vi "NanotecSMCPDDriver.create write string.vi"(1 "contollerID":i32, 3 "commandString":string, 5 "error in (no error)":errorcluster) -> (15 "writeString":string, 17 "expextedReturnString":string, 19 "error out":errorcluster)   [LabVIEW 2014, in "NanotecSMCPDDriver.lvlib"]
doc: "Composes the string, that will be written to the serial interface.\n\nTo access an individual controller, the controllerID must be in the range 1..254.\nTo select all controllers, the controllerID must equal -2."
uses:
  NanotecSMCPDDriver.lvlib
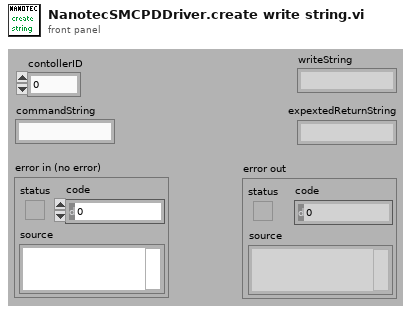
[diagram p1: front panel]
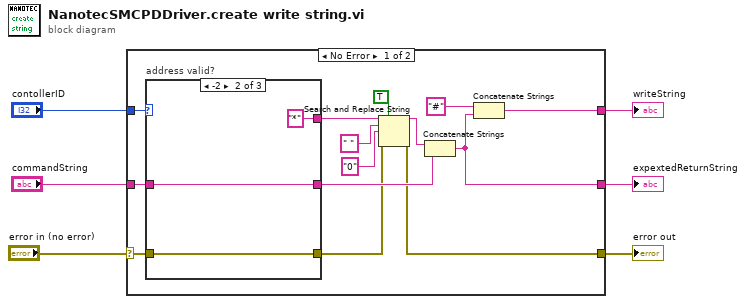
[diagram p0: block diagram]
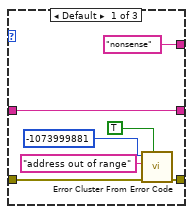
[diagram p2: hidden frame]
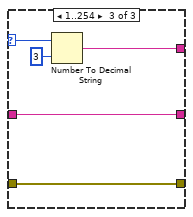
[diagram p3: hidden frame]
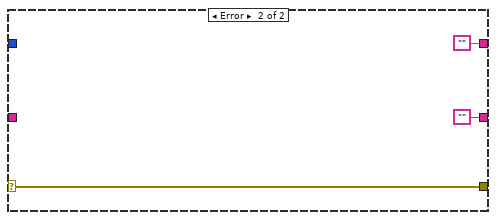
[diagram p4: hidden frame]
diagram:
  n1 = case shown="No Error" "error in (no error)" {
    selector: "error in (no error)" -> [w11 w38]
    tunnel: [w20 "" ("Empty String Constant")] -> w6
    tunnel: [w19 "" ("Empty String Constant")] -> w5
    tunnel: "commandString" -> [w10 _]
    tunnel: "contollerID" -> [w12 _]
    tunnel: [w8 w38] -> w2
    frame No Error {
      n2 = case "address valid?" shown="-2" w12 {
        selector: w12 -> [_ _ w33]
        tunnel: ["nonsense" "*" w35] -> w13
        tunnel: w11 -> [w26 w29 w32]
        tunnel: [w22 w29 w32] -> w7
        tunnel: w10 -> [w21 w28 w31]
        tunnel: [w21 w28 w31] -> w9
        frame Default {
          n3 = call <vilib>:"Error Cluster From Error Code.vi"("show call chain? (False)"=TRUE, "error in (no error)"=w26, "error message (\"\")"="address out of range", "error code (0)"=-1073999881) -> ("error out"=w22:errorcluster)  [unwired: 5 in]
        }
        frame -2 {
        }
        frame 1..254 {
          n4 = Number To Decimal String(number=w33, width (-)=i16 3) -> (decimal integer string=w35:string)
        }
      }
      n5 = Search and Replace String(replace all?=TRUE ("replace all? (F)"), input string=w13, search string=" ", replace string="0" ("replace string (\"\")"), error in=w7) -> (result string=w17:string, error out=w8:errorcluster)  [unwired: 3 in, 2 out]
      n6 = Concatenate Strings(w17, w9) -> (w20:string)
      n7 = Concatenate Strings("#" ("string"), w20) -> (w19:string)
    }
    frame Error {
    }
  }
  "expextedReturnString" <- w6
  "writeString" <- w5
  "error out" <- w2
